vi "TP 4.2.vi"() -> ()   [LabVIEW 2013]
uses:
  <vilib>/sound2/lvsound2.llb/Sound Input Read (DBL).vi
panel:
  out "Correlacion":dbl
  in  "Frecuencia":dbl=1000.0
  out "Umbral":bool
  in  "Cluster":T1={"Sample rate"=44100.0, "N channels"=1.0, " Bits/Sample"=16.0}
  out "Waveform Graph":dbl[](graph)
  in  "Buffer de lectura":dbl=11025.0
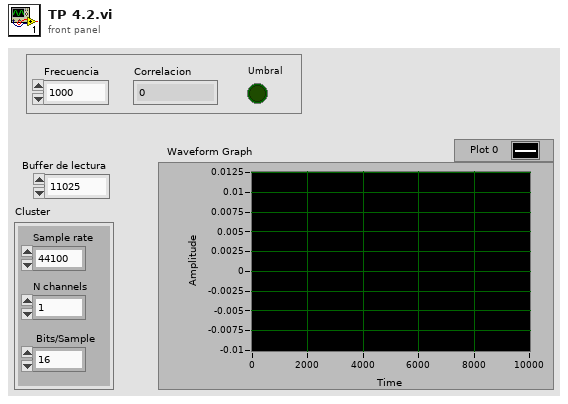
[diagram p1: front panel]
types:
  T1 = cluster{"Sample rate":dbl, "N channels":dbl, " Bits/Sample":dbl}
  T2 = typedef "Sound Input Task ID.ctl" = u32
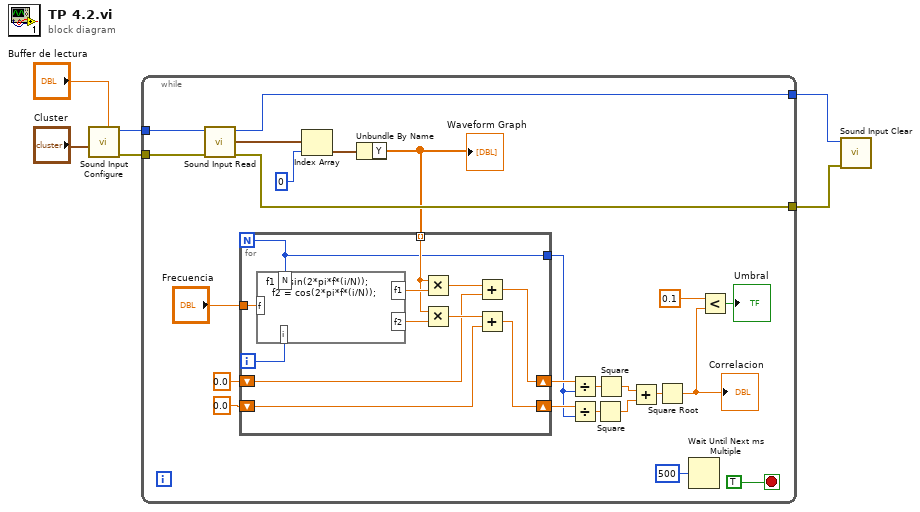
[diagram p0: block diagram]
diagram:
  n1 = call <vilib>:"Sound Input Configure.vi"("number of samples/ch"="Buffer de lectura", "sound format"="Cluster") -> ("error out"=w4:errorcluster, "task ID"=w5:T2)  [unwired: 8 in]
  n2 = while {
    tunnel: w5 -> [w27]
    tunnel: w4 -> [w26]
    tunnel: [w25] -> w2
    tunnel: [w24] -> w1
    stop <- TRUE stop-if-true
    n3 = call-poly <vilib>:"Sound Input Read.vi"("error in (no error)"=w26, "task ID"=w27) -> ("error out"=w24:errorcluster, "data"=w30:waveform(dbl)[], "task ID out"=w25:T2)  [unwired: 7 in]
    n4 = Index Array(array=w30, index=0) -> (element=w28:waveform(dbl))
    n5 = Unbundle By Name(w28) -> ("Y"=w21:dbl[])
    "Waveform Graph" <- w21
    n6 = for {
      N -> [w31]
      tunnel: "Frecuencia" -> [w41]
      tunnel: w21 -> [w38] mode=indexing
      shift-right: [w35] -> w12
      shift-left: 0.0 -> [w32]
      shift-right: [w34] -> w13
      shift-left: 0.0 -> [w33]
      tunnel: [w31] -> w11
      i -> [w42]
      n7 = formula code="f1 = sin(2*pi*f*(i/N));\n  f2 = cos(2*pi*f*(i/N));"("f"=w41, "N"=w31, "i"=w42) -> ("f1"=w40:dbl, "f2"=w39:dbl)
      n8 = Multiply(x=w38, y=w40) -> (x*y=w37:dbl)
      n9 = Multiply(x=w38, y=w39) -> (x*y=w36:dbl)
      n10 = Add(x=w37, y=w32) -> (x+y=w35:dbl)
      n11 = Add(x=w36, y=w33) -> (x+y=w34:dbl)
    }
    n12 = Divide(x=w12, y=w11) -> (x/y=w17:dbl)
    n13 = Divide(x=w13, y=w11) -> (x/y=w18:dbl)
    n14 = Square(x=w18) -> (x^2=w15:dbl)
    n15 = Square(x=w17) -> (x^2=w16:dbl)
    n16 = Add(x=w16, y=w15) -> (x+y=w14:dbl)
    n17 = Square Root(x=w14) -> (sqrt(x)=w9:dbl)
    "Correlacion" <- w9
    n18 = Wait Until Next ms Multiple(millisecond multiple=u32 500) -> ()  [unwired: 1 out]
    n19 = Less?(x=0.1, y=w9) -> (x < y?=→"Umbral":bool)
  }
  n20 = call <vilib>:"Sound Input Clear.vi"("error in (no error)"=w1, "task ID"=w2) -> ()  [unwired: 9 in, 1 out]
